vi "SyncLoop.vi"(8 "error in (no error)":errorcluster, 11 "NiPxi6683H in":refnum<class "NiPxi6683H.lvclass">) -> (0 "error out":errorcluster, 1 "Locked":bool, 2 "Time Ref Offset (ns)":dbl format="%#_12f", 3 "NiPxi6683H out":refnum<class "NiPxi6683H.lvclass">, 4 "Lost Lock":bool, 6 "ObtainLock":bool)   [LabVIEW 2014, in "SyncPlugins.lvlib" / "NiPxi6683H.lvclass"]
uses:
  NiPxi6683H.lvclass
  SyncPluginBase/SyncPluginBase.lvclass/SyncPluginBase.ctl
  NiPxi6682/NiPxi6682.lvclass/NiPxi6682.ctl
  SyncPluginBase/Accessors/Write Locked.vi
  SyncPluginBase/Accessors/Write PPSTime.vi
  NiPxi6682/Accessors/Read NiSyncHandle.vi
  NiPxi6682/Accessors/Read 1PPS.vi
  NiPxi6682/Accessors/Read SysRef.vi
  SyncPluginBase/Accessors/Read Run.vi
  SyncPluginBase/Accessors/Read Locked.vi
  <instrlib>/niSync/niSync.llb/niSync Read Trigger Time Stamp (Single).vi
  <resource>/objmgr/niflexriosae.rc
panel:
  out "time stamp out":timestamp
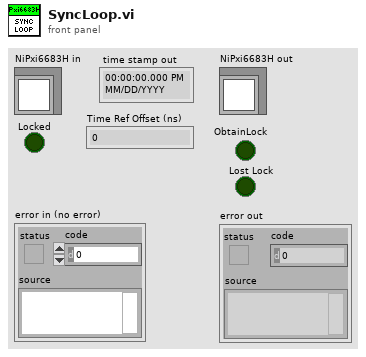
[diagram p1: front panel]
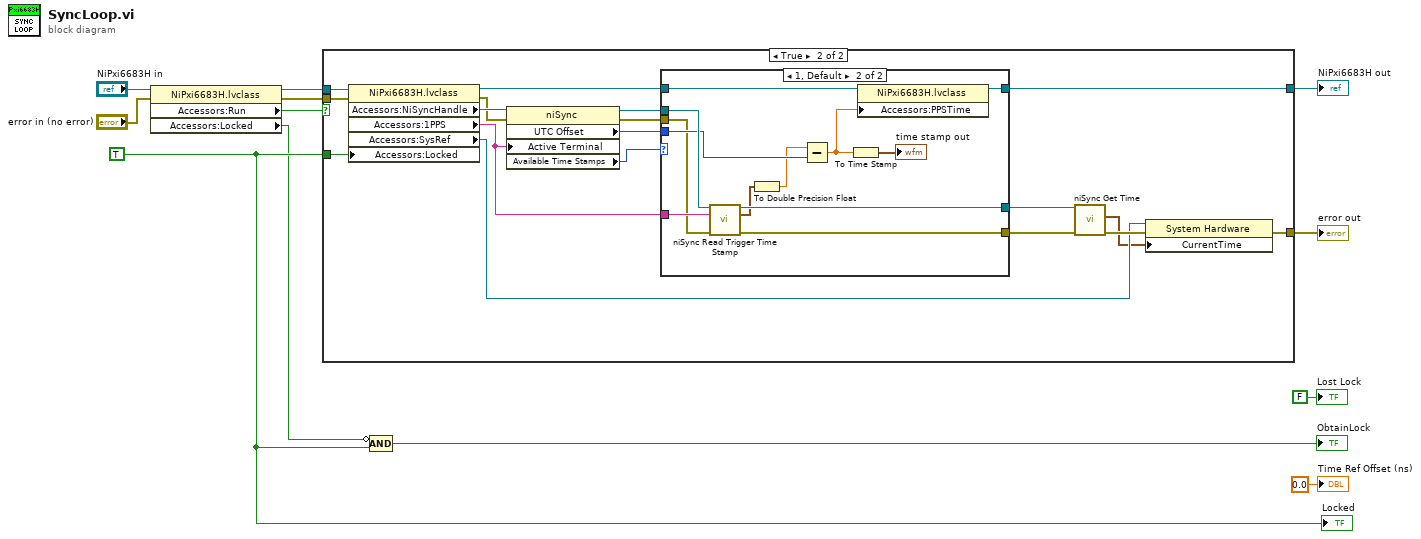
[diagram p0: block diagram]
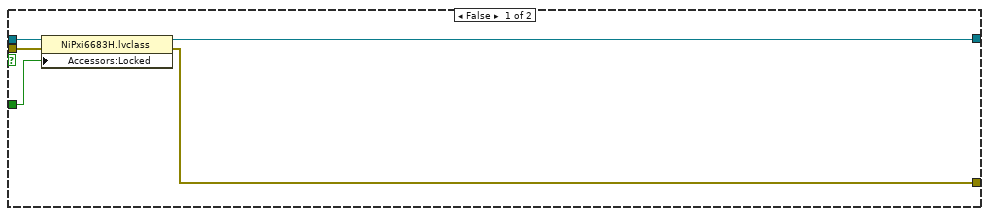
[diagram p2: hidden frame]
diagram:
  w5 = TRUE ("Locked")
  n1 = property class="NiPxi6683H.lvclass"(reference="NiPxi6683H in", error in="error in (no error)") -> (reference out=w10:refnum<class "NiPxi6683H.lvclass">, error out=w2:errorcluster, "Accessors:Run"=w11:bool, "Accessors:Locked"=w3:bool)
  n2 = case shown="True" w11 {
    tunnel: w10 -> [w17 w35]
    tunnel: [w16 w32] -> w9
    tunnel: [w13 w26] -> w8
    tunnel: w5 -> [w15 w23]
    tunnel: w2 -> [w14 w22]
    frame False {
      n3 = property class="NiPxi6683H.lvclass"(reference=w17, error in=w14, "Accessors:Locked"=w15) -> (reference out=w16:refnum<class "NiPxi6683H.lvclass">, error out=w13:errorcluster)
    }
    frame True {
      n4 = property class="NiPxi6683H.lvclass"(reference=w35, error in=w22, "Accessors:Locked"=w23) -> (reference out=w33:refnum<class "NiPxi6683H.lvclass">, error out=w21:errorcluster, "Accessors:NiSyncHandle"=w34:refnum<k15>, "Accessors:1PPS"=w18:tag, "Accessors:SysRef"=w25:refnum<k20>)
      n5 = property class="niSync"(reference=w34, error in=w21, "Active Terminal"=w18) -> (reference out=w30:refnum<k15>, error out=w20:errorcluster, "UTC Offset"=w28:i32, "Available Time Stamps"=w19:i32)
      n6 = case shown="1, Default" w19 {
        tunnel: w33 -> [w38 w50]
        tunnel: [w38 w49] -> w32
        tunnel: [w37 w48] -> w31
        tunnel: w30 -> [w36 w47]
        tunnel: [w36 w46] -> w29
        tunnel: w28 -> [_ w44]
        tunnel: w18 -> [_ w41]
        tunnel: w20 -> [w37 w39]
        frame 0 {
        }
        frame 1, Default {
          n7 = call-poly <instrlib>:"niSync Read Trigger Time Stamp.vi"("instrument handle"=w47, "terminal"=w41, "error in (no error)"=w39) -> ("instrument handle out"=w46:refnum<k15>, "time stamp out"=w42:timestamp, "error out"=w48:errorcluster)  [unwired: 9 in, 1 out]
          n8 = To Double Precision Float(number=w42) -> (double precision float=w43:dbl)
          n9 = Subtract(x=w43, y=w44) -> (x-y=w40:dbl)
          n10 = To Time Stamp(1:w40) -> (0:→"time stamp out":timestamp)
          n11 = property class="NiPxi6683H.lvclass"(reference=w50, "Accessors:PPSTime"=w40) -> (reference out=w49:refnum<class "NiPxi6683H.lvclass">)  [unwired: 1 in, 1 out]
        }
      }
      n12 = call <instrlib>:"niSync Get Time.vi"("error in (no error)"=w31, "instrument handle"=w29) -> ("error out"=w27:errorcluster, "time"=w24:timestamp)  [unwired: 5 in, 1 out]
      n13 = property class="System Hardware"(reference=w25, error in=w27, "CurrentTime"=w24) -> (error out=w26:errorcluster)  [unwired: 1 out]
    }
  }
  "error out" <- w8
  "NiPxi6683H out" <- w9
  n14 = Compound Arithmetic op=AND(invert w3, w5) -> (→"ObtainLock":bool)
  "Locked" <- w5
  "Time Ref Offset (ns)" <- 0.0 ("Time Ref Offset (ns)")
  "Lost Lock" <- FALSE ("Lost Lock")
